vi "Analyze Data.vi"(8 "error in":errorcluster, 11 "nCRD in":refnum<class "nCRD.lvclass">) -> (0 "error out":errorcluster, 3 "nCRD out":refnum<class "nCRD.lvclass">)   [LabVIEW 2014, in "nCRD.lvclass"]
doc: "Analyze Data takes the stored ringdown data (1000 shots per cell) and:\n1) Calculates the ringdown decay constant tau\n2) Averages tau0 data as necessary\n3) Corrects the tau data for Rayleigh scattering\n4) Stores a 1-D array of taus returned on a 1 kHz basis (8k taus) if a jump drive (U:) is connected\n5) Flattens the data into a string and stuffs the string into the <b>data</b> shared variable for display on the UI.\n\nThis VI will not be called if the data is not \"good\" (that is, if an error was thrown in the <B>Get Data</B> routine. If an error is thrown while the data is being retrieved, then the data will not be sent to the UI."
uses:
  nCRD.lvclass
  Reusable/CRDS/Main/CRDS.lvclass/CRDS.ctl
  nCRD.lvclass/nCRD.ctl
  Data/Nicholas Data.lvclass/Nicholas Data.ctl
  Reusable/CRDS/Main/Read Laser Data.vi
  Accessors/Read Data DVR.vi
  Data/Write CRDS.vi
  Reusable/CRDS/Main/Read Data.vi
  Reusable/CRDS/Main/CRDS.lvclass
  Reusable/CRDS/Data/Main/CRDS Data.lvclass
  Data/Nicholas Data.lvclass
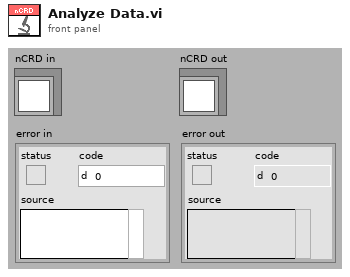
[diagram p1: front panel]
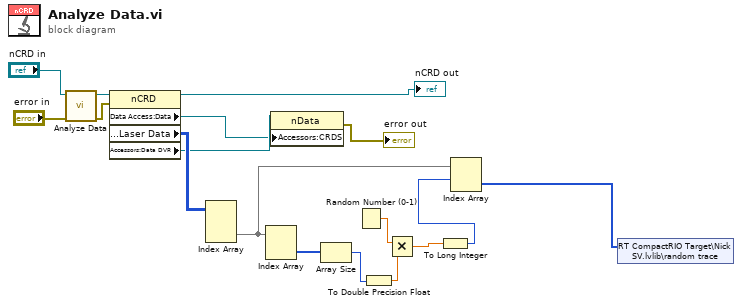
[diagram p0: block diagram]
diagram:
  n1 = call-parent "Analyze Data.vi"("error in"="error in", "CRDS in"="nCRD in") -> ("error out"=w13:errorcluster, "CRDS out"=w14:refnum<class "nCRD.lvclass">)  [unwired: 8 in]
  n2 = property class="nCRD"(reference=w14, error in=w13) -> (reference out=→"nCRD out":refnum<class "nCRD.lvclass">, "Data Access:Data"=w2:refnum<class "CRDS Data.lvclass">, "Data Access:Laser Data"=w12:i16[][][], "Accessors:Data DVR"=w3:refnum<data-value>)  [unwired: 1 out]
  n3 = Index Array(array=w12) -> (element=w6:i16[][])  [unwired: 3 in]
  n4 = Index Array(array=w6) -> (element=w11:i16[])  [unwired: 2 in]
  n5 = property class="nData"(reference=w3, "Accessors:CRDS"=w2) -> (error out=→"error out":errorcluster)  [unwired: 1 in, 1 out]
  n6 = Array Size(array=w11) -> (size(s)=w8:i32)
  n7 = Random Number (0-1)() -> (number: 0 to 1=w10:dbl)
  n8 = To Double Precision Float(number=w8) -> (double precision float=w7:dbl)
  n9 = Multiply(x=w10, y=w7) -> (x*y=w9:dbl)
  n10 = To Long Integer(number=w9) -> (32bit integer=w5:i32)
  n11 = Index Array(array=w6, index (row)=w5) -> (element=w4:i16[])  [unwired: 1 in]
  n12 = shared-variable "RT CompactRIO Target\\Nick SV.lvlib\\random trace"(w4) -> ()  [unwired: 1 in, 1 out]
